vi "getMissingCellPolicy.vi"(8 "error in (no error)":errorcluster) -> (0 "error out":errorcluster, 3 "CREATE_NULL_AS_BLANK":refnum<k24>)   [LabVIEW 2017, in "LabVIEW NPOI.lvlib" / "MS-Excel.lvclass"]
uses:
  MS-Excel.lvclass
  D:/Benjamin/Documents/Perso/Code/WC/LabVIEW_NPOI/lib/NPOI 2.1.1/NPOI.dll
  lib/NPOI 2.1.1/NPOI.dll
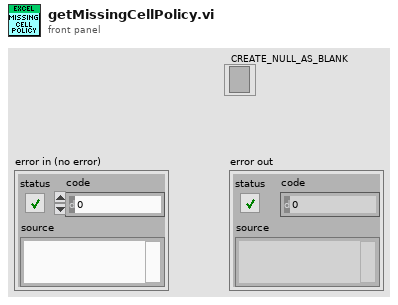
[diagram p1: front panel]
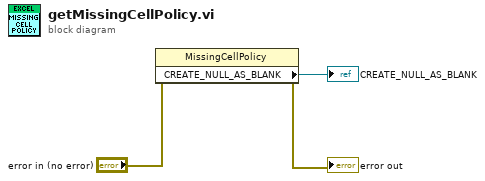
[diagram p0: block diagram]
diagram:
  n1 = property class="MissingCellPolicy"(error in="error in (no error)") -> (error out=→"error out":errorcluster, "CREATE_NULL_AS_BLANK"=→"CREATE_NULL_AS_BLANK":refnum<k24>)  [unwired: 1 in, 1 out]
